vi "Check For MD5 Change.vi"(8 "error in":errorcluster, 11 "configuration files page data":T1 {"custom device ref" format="%.0x"}) -> (0 "error out":errorcluster, 2 "MD5 change?":bool, 3 "configuration files page data out":T1 {"custom device ref" format="%.0x"})   [LabVIEW 2020, in "AIM ARINC 429 System Explorer.lvlib" / "Implementation.lvlib"]
uses:
  Implementation.lvlib
  <vilib>/NI VeriStand/Custom Device API/Custom Device Item Ref.ctl
  <vilib>/NI VeriStand/Custom Device API/Custom Device API.lvlib
  Types/Browse Button.ctl
  Types/Path Control.ctl
  Types/Configuration Files Page Data.ctl
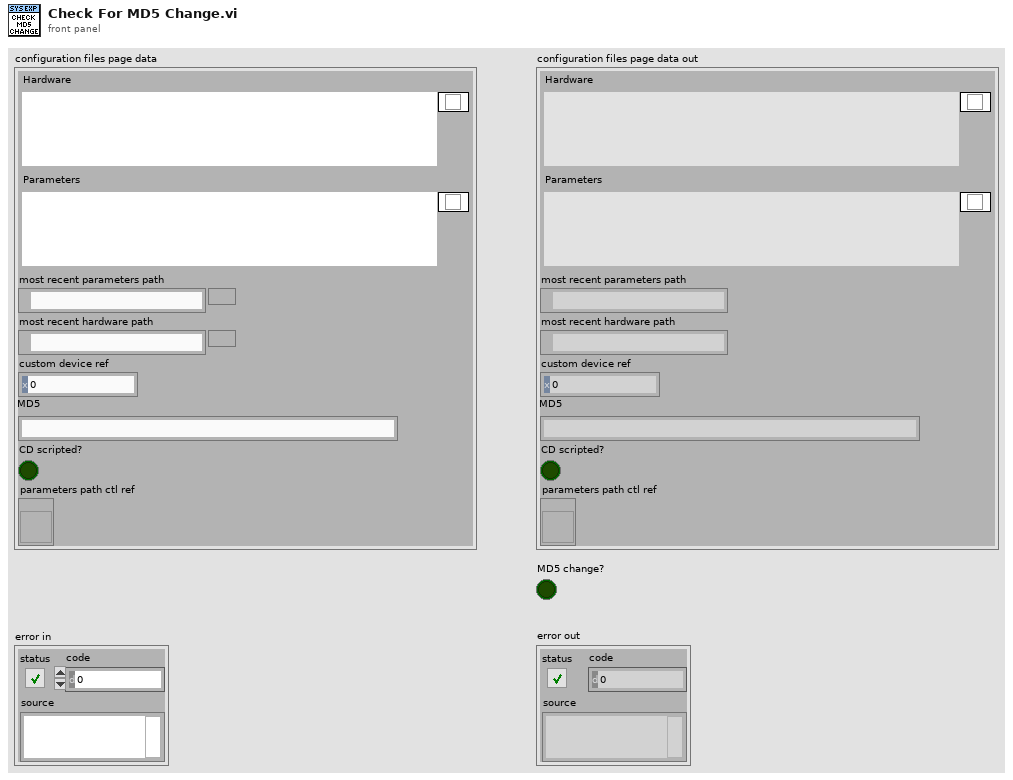
[diagram p1: front panel]
types:
  T1 = typedef "AIM ARINC 429 System Explorer.lvlib/Implementation.lvlib/Configuration Files Page Data.ctl" = cluster{"Hardware":T2, "Parameters":T2, "most recent parameters path":path, "most recent hardware path":path, "custom device ref":T4, "MD5":string, "CD scripted?":bool, "parameters path ctl ref":refnum<vi>}
  T2 = typedef "AIM ARINC 429 System Explorer.lvlib/Implementation.lvlib/Path Control.ctl" = cluster{"file path":path, "Browse":T3}
  T3 = typedef "AIM ARINC 429 System Explorer.lvlib/Implementation.lvlib/Browse Button.ctl" = bool
  T4 = typedef "Custom Device API.lvlib/Custom Device Item Ref.ctl" = u64
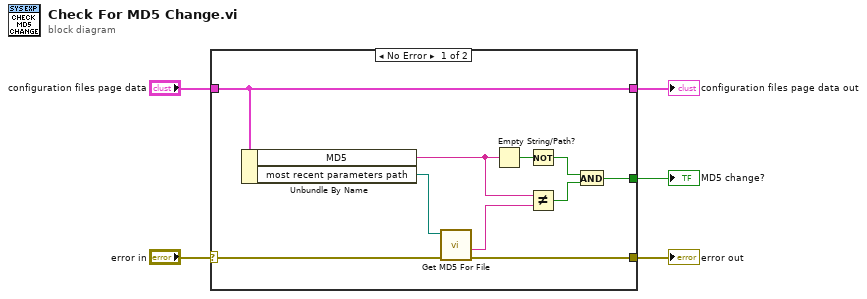
[diagram p0: block diagram]
diagram:
  n1 = case shown="No Error" "error in" {
    selector: "error in" -> [w14 w17]
    tunnel: [w11 w17] -> w4
    tunnel: "configuration files page data" -> [w6 w16]
    tunnel: [w6 w16] -> w2
    tunnel: [w7 _] -> w1
    frame No Error {
      n2 = Unbundle By Name(w6) -> ("MD5"=w12:string, "most recent parameters path"=w15:path)
      n3 = call "Get MD5 For File.vi"("error in"=w14, "path"=w15) -> ("error out"=w11:errorcluster, "MD5"=w13:string)  [unwired: 8 in]
      n4 = Empty String/Path?(string/path=w12) -> (empty?=w10:bool)
      n5 = Not(x=w10) -> (.not. x?=w8:bool)
      n6 = Not Equal?(x=w12, y=w13) -> (x != y?=w9:bool)
      n7 = And(x=w8, y=w9) -> (x .and. y?=w7:bool)
    }
    frame Error {
    }
  }
  "error out" <- w4
  "configuration files page data out" <- w2
  "MD5 change?" <- w1
